vi "Secure Server Connection.vi"(0 "TCP connection":refnum<k5>, 1 "private key":u8[](array[numeric]), 3 "certificate chain":cluster{"certificate":u8[]}[](array[cluster]), 5 "error in":errorcluster, 9 "load OS trusted CAs?":bool, 10 "timeout (25000 ms)":i32=25000) -> (14 "TCP connection out":refnum<k5>, 18 "server certificate chain":cluster{"certificate":u8[]}[](array[cluster]), 19 "error out":errorcluster)   [LabVIEW 2021, in "LV WebSockets.lvlib"]
doc: "Configures and negotiates a TLS server connection"
uses:
  LV WebSockets.lvlib
  <vilib>/Utility/error.llb/Error Cluster From Error Code.vi
  <vilib>/ErrorRing/Error Ring.xnode
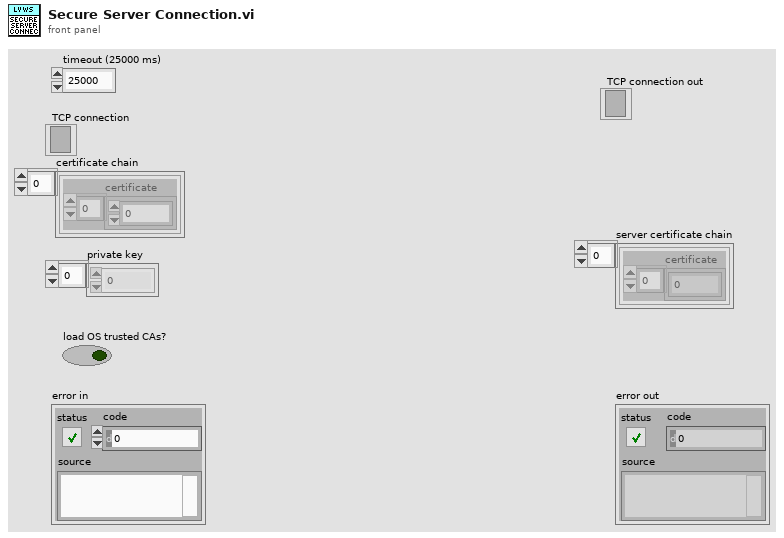
[diagram p1: front panel]
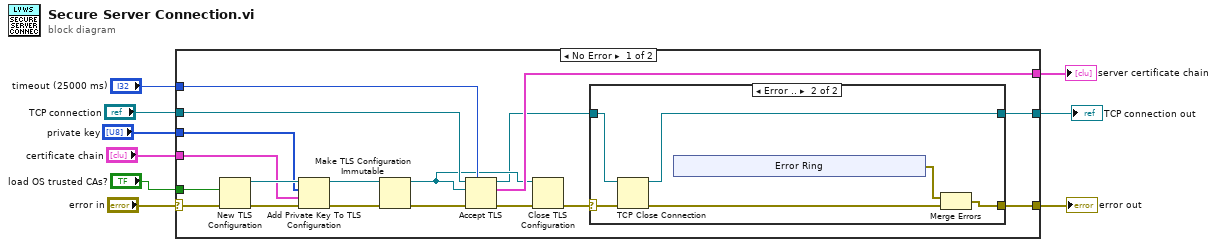
[diagram p0: block diagram]
diagram:
  n1 = case shown="No Error" "error in" {
    selector: "error in" -> [w25 w41]
    tunnel: "timeout (25000 ms)" -> [w27 _]
    tunnel: [w26 w42] -> w8
    tunnel: "load OS trusted CAs?" -> [w24 _]
    tunnel: [w10 w41] -> w5
    tunnel: "TCP connection" -> [w17 w43]
    tunnel: [w11 w43] -> w3
    tunnel: "private key" -> [w16 _]
    tunnel: "certificate chain" -> [w15 w42]
    frame No Error {
      n2 = New TLS Configuration(8:w25, 10:w24) -> (0:w22:errorcluster, 3:w20:refnum<k36>)
      n3 = Add Private Key To TLS Configuration(8:w22, 9:w15, 10:w16, 11:w20) -> (0:w21:errorcluster, 3:w19:refnum<k36>)
      n4 = Make TLS Configuration Immutable(8:w21, 11:w19) -> (0:w18:errorcluster, 3:w14:refnum<k36>)
      n5 = Accept TLS(7:w27, 8:w18, 10:w14, 11:w17) -> (0:w23:errorcluster, 2:w26:cluster{"certificate":u8[]}[], 3:w12:refnum<k5>)
      n6 = Close TLS Configuration(8:w23, 11:w14) -> (0:w13:errorcluster)
      n7 = case shown="Error .." w13 {
        selector: w13 -> [w28 w35]
        tunnel: w12 -> [w29 w34]
        tunnel: [w29 w33] -> w11
        tunnel: [w28 w30] -> w10
        frame No Error {
        }
        frame Error {
          n8 = TCP Close Connection(connection ID=w34, error in (no error)=w35) -> (connection ID out=w33:refnum<k5>, error out=w31:errorcluster)  [unwired: 1 in]
          n9 = xnode ("Error Ring")() -> ("error out"=w32:errorcluster)
          n10 = Merge Errors(w32, w31) -> (w30:errorcluster)
        }
      }
    }
    frame Error {
    }
  }
  "server certificate chain" <- w8
  "error out" <- w5
  "TCP connection out" <- w3
